vi "Histogram Test.vi"() -> ()   [LabVIEW 2012]
panel:
  out "x^y":dbl
  in  "Histogram Bin":string(combo)
  in  "Stop Delay  (ns)":i16 min=0 max=1008 step=16
  out "Waveform Graph":cluster{i16, dbl, "Array":i64[]}(graph)
  in  "Start Measurement":bool
  out "Single Count Channel4":i64
  out "Single Count Channel3":i64
  out "Single Count Channel2":i64
  out "Single Count Channel1":i64
  out "Exposition time (ms)":i64
  out "Measurement index":i64
  out "Start OK":bool
  in  "Exit":bool
  in  "Single Count Enable":T1
  in  "Channel4 Pulse Front":string
  in  "Channel4 Threshold Voltage (mV)":i32
  in  "Channel3 Pulse Front":string
  in  "Channel3 Threshold Voltage (mV)":i32
  in  "Channel2 Pulse Front":string
  in  "Channel2 Threshold Voltage (mV)":i32
  in  "Channel1 Pulse Front":string(combo)
  in  "Channel1 Threshold Voltage (mV)":i32 min=0 max=5000 step=10
  in  "Exposition Time (ms)":i64
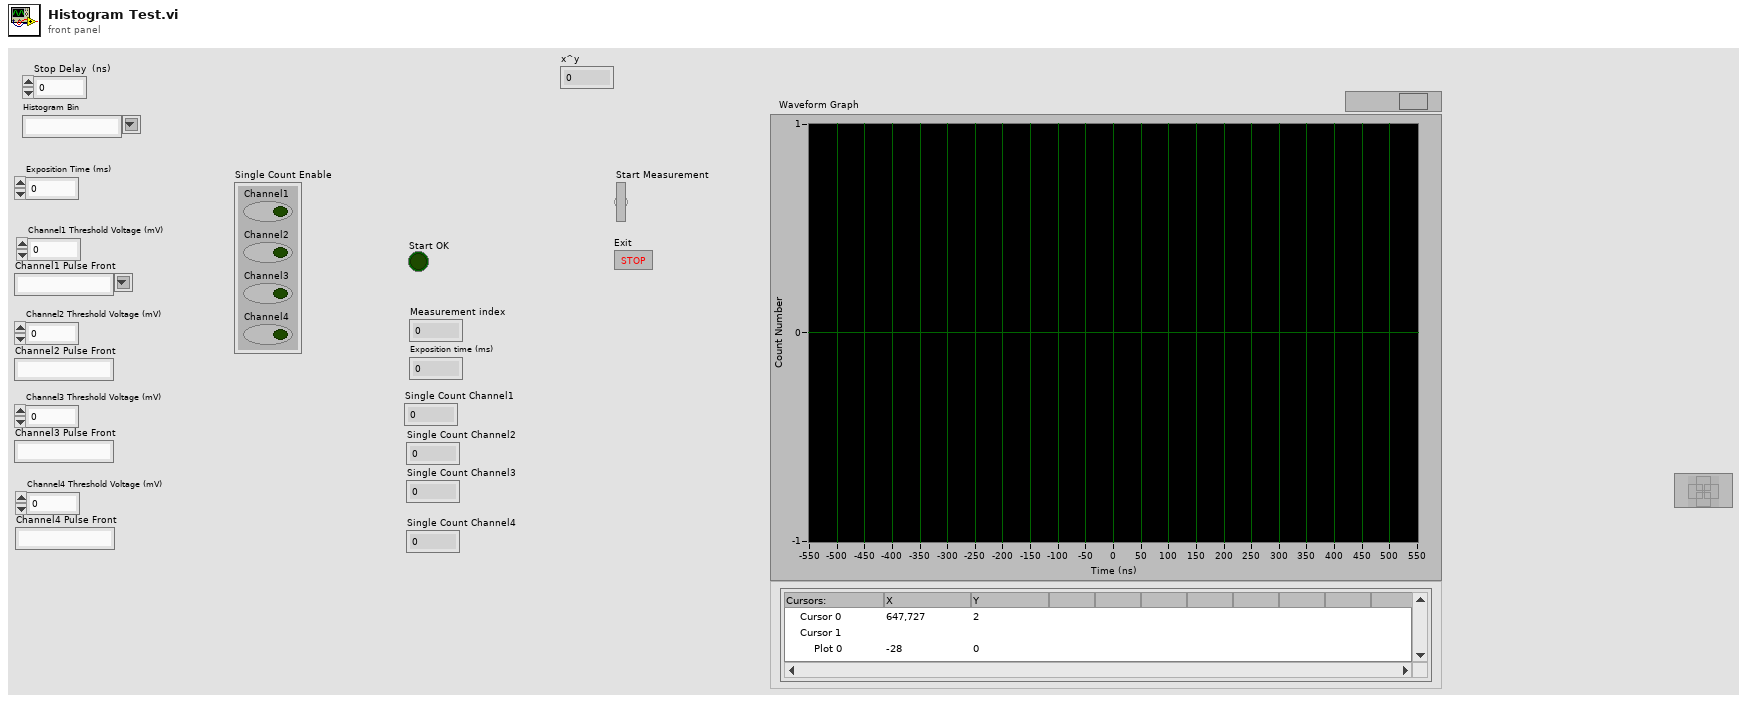
[diagram p1: front panel]
types:
  T1 = cluster{"Channel1":bool, "Channel2":bool, "Channel3":bool, "Channel4":bool}
  T2 = cluster{"[0]":i64, "Channel1 Threshold Voltage (mV)":i32, "Channel1 Pulse Front":string, "Channel2 Threshold Voltage (mV)":i32, "Channel2 Pulse Front":string, "Channel3 Threshold Voltage (mV)":i32, "Channel3 Pulse Front ":string, "Channel4 Threshold Voltage (mV)":i32, "Channel4 Pulse Front ":string, "Single Count Enable":cluster{"Channel1":bool, "Channel2":bool, "Channel3":bool, "Channel4":bool}, "Single Count Max":i32, "Sum Count Enable":cluster{"Channel1":bool, "Channel2":bool, "Channel3":bool, "Channel4":bool}, "Sum Count Max":i32, "Start-Stop1 Multyplex":cluster{"Stop Channel":string, "Start Channel":string}, "Stop Delay 1 (ns)":i16, "Window Length 1 (ns)":i32, "Window Offset 1 (ns) ":i32, "Conditional Correlation 1":string, "Histogram Bin 1":string, "Histogram Start 1 (ns) ":i32, "Start-Stop2 Multyplex ":cluster{"Stop Channel":string, "Start Channel":string}, "Stop Delay 2 (ns)":i16, "Window Length 2 (ns) ":i32, "Window Offset 2 (ns) ":i32, "Conditional Correlation 2":string, "Histogram Bin 2":string, "Histogram Start 2 (ns)  ":i32, "Start-Stop3 Multyplex":cluster{"Stop Channel":string, "Start Channel":string}, "Stop Delay 3 (ns)":i16, "Window Length 3 (ns) ":i32, "Window Offset 3 (ns) ":i32, "Conditional Correlation 3":string, "Histogram Bin 3":string, "Histogram Start 3 (ns) ":i32, "Start-Stop4 Multyplex":cluster{"Stop Channel":string, "Start Channel":string}, "Stop Delay 4 (ns)":i16, "Window Length 4 (ns)  ":i32, "Window Offset 4 (ns) ":i32, "Conditional Correlation 4":string, "Histogram Bin 4":string, "Histogram Start 4 (ns)  ":i32, "Coincidence Count Enable":cluster{"Start-Stop1":bool, "Start-Stop2":bool, "Start-Stop3":bool, "Start-Stop4":bool}, "Coincidence Count Max":i32, "Coincidence Sum Enable":cluster{"Start-Stop1":bool, "Start-Stop2":bool, "Start-Stop3":bool, "Start-Stop4":bool}, "Coincidence Sum Max":i32, "Output Channel Enable":cluster{"Channel1":bool, "Channel2":bool, "Channel3":bool, "Channel4":bool}, "Output Channel Inversion":cluster{"Channel1":bool, "Channel2":bool, "Channel3":bool, "Channel4":bool, "Output":bool}}
  T3 = cluster{"Going":bool, "Iinterrupted":bool, "Timer stop":bool, "Single count stop Ch1":bool, "Single count stop Ch2":bool, "Single count stop Ch3":bool, "Single count stop Ch4":bool, "Sum count stop":bool, "Coincidence count stop SS1":bool, "Coincidence count stop SS2":bool, "Coincidence count stop SS3":bool, "Coincidence count stop SS4":bool, "Coincidence sum count stop":bool, "Reserved":bool, "Correlator is not initialised":bool, "Internal error":bool}
  T4 = cluster{"Measurement index":i64, "Exposition time (ms)":i64, "Single Count Channel1":i64, "Single Count Channel2":i64, "Single Count Channel3":i64, "Single Count Channel4":i64, "Sum Single Count":i64, "Coincidence Count SS1":i64, "Coincidence Count SS2":i64, "Coincidence Count SS4":i64, "Coincidence Count SS5":i64, "Sum Coincidence Count":i64}
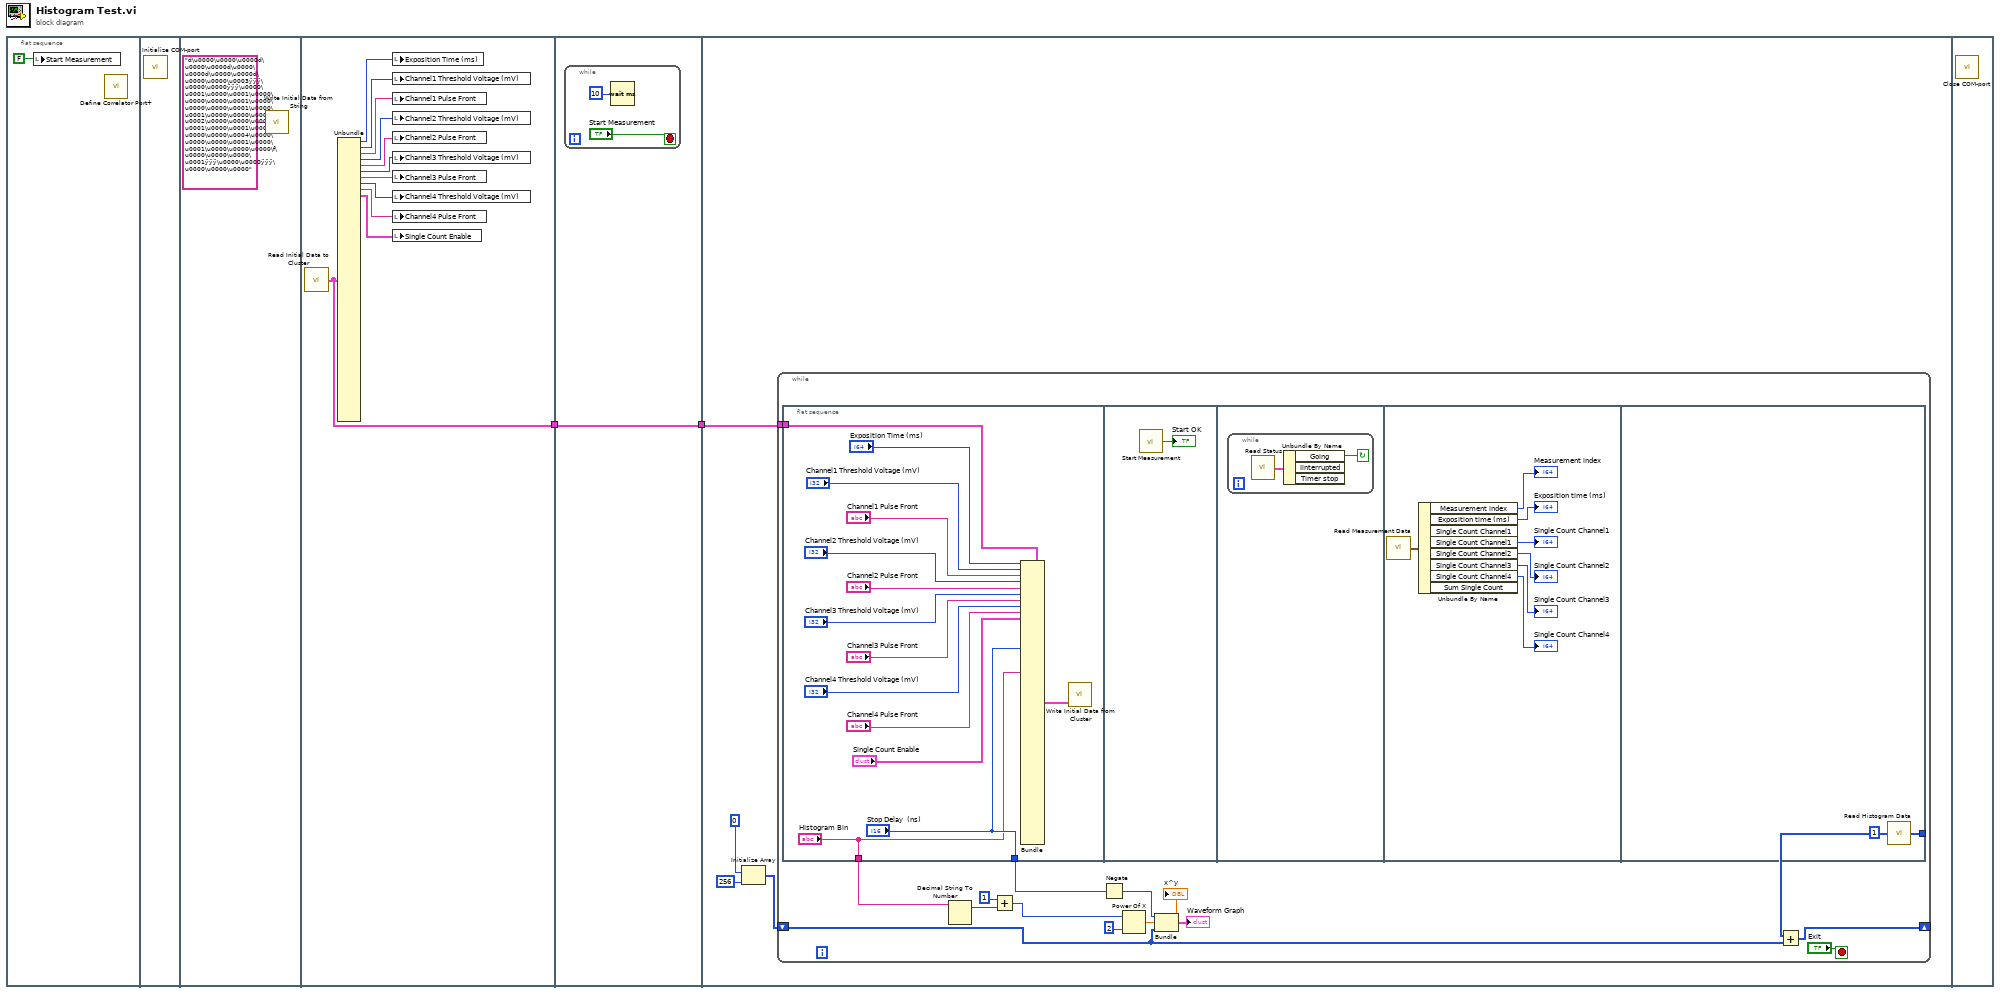
[diagram p0: block diagram]
diagram:
  n1 = flat-sequence {
    tunnel: [w15] -> w2
    tunnel: w2 -> [w16]
    tunnel: [w16] -> w1
    tunnel: w1 -> [w22]
    frame #0 {
      n2 = local write "Start Measurement"(FALSE ("Start Measurement")) -> ()
      n3 = call "Define Correlator Port+.vi"() -> ()  [unwired: 3 in]
    }
    frame #1 {
      n4 = call "Initialize COM-port.vi"() -> ()  [unwired: 4 in]
    }
    frame #2 {
      n5 = call "Write Initial Data from String.vi"("Data"="d\u0000\u0000\u0000d\u0000\u0000d\u0000\u0000d\u0000\u0000d\u0000\u0000\u0003ÿÿÿ\u0000\u0000ÿÿÿ\u0000\u0001\u0000\u0001\u0000\u0000\u0000\u0001\u0000\u0000\u0000\u0001\u0000\u0001\u0000\u0000\u0000\u0002\u0000\u0000\u0000\u0001\u0000\u0001\u0000\u0000\u0000\u0004\u0000\u0000\u0000\u0001\u0000\u0001\u0000\u0000\u0000\f\u0000\u0000\u0000\u0001ÿÿÿ\u0000\u0000ÿÿÿ\u0000\u0000\u0000") -> ()  [unwired: 1 out]
    }
    frame #3 {
      n6 = call "Read Initial Data to Cluster.vi"() -> ("Correlator Initial Data 2"=w15:T2)  [unwired: 2 in]
      n7 = Unbundle(w15) -> ("[0]"=w14:i64, "Channel1 Threshold Voltage (mV)"=w13:i32, "Channel1 Pulse Front"=w12:string, "Channel2 Threshold Voltage (mV)"=w11:i32, "Channel2 Pulse Front"=w10:string, "Channel3 Threshold Voltage (mV)"=w9:i32, "Channel3 Pulse Front"=w8:string, "Channel4 Threshold Voltage (mV)"=w7:i32, "Channel4 Pulse Front"=w6:string, "Single Count Enable"=w5:T1)  [unwired: 37 out]
      n8 = local write "Exposition Time (ms)"(w14) -> ()
      n9 = local write "Channel1 Threshold Voltage (mV)"(w13) -> ()
      n10 = local write "Channel1 Pulse Front"(w12) -> ()
      n11 = local write "Channel2 Threshold Voltage (mV)"(w11) -> ()
      n12 = local write "Channel2 Pulse Front"(w10) -> ()
      n13 = local write "Channel3 Threshold Voltage (mV)"(w9) -> ()
      n14 = local write "Channel3 Pulse Front"(w8) -> ()
      n15 = local write "Channel4 Threshold Voltage (mV)"(w7) -> ()
      n16 = local write "Channel4 Pulse Front"(w6) -> ()
      n17 = local write "Single Count Enable"(w5) -> ()
    }
    frame #4 {
      n18 = while {
        stop <- "Start Measurement" stop-if-true
        n19 = Wait (ms)(milliseconds to wait=u32 10) -> ()  [unwired: 1 out]
      }
    }
    frame #5 {
      n20 = Initialize Array(i64 0 ("Value"), 256 ("dimension size")) -> (w21:i64[])
      n21 = while {
        tunnel: w22 -> [w35]
        shift-right: [w33] -> _
        shift-left: w21 -> [w23]
        stop <- "Exit" stop-if-true
        n22 = flat-sequence {
          tunnel: w35 -> [w42]
          tunnel: ["Stop Delay  (ns)"] -> w31
          tunnel: ["Histogram Bin"] -> w29
          tunnel: [w61] -> w34
          frame #0 {
            n23 = Bundle(cluster=w42, "[0]"="Exposition Time (ms)", "Channel1 Threshold Voltage (mV)"="Channel1 Threshold Voltage (mV)", "Channel1 Pulse Front"="Channel1 Pulse Front", "Channel2 Threshold Voltage (mV)"="Channel2 Threshold Voltage (mV)", "Channel2 Pulse Front"="Channel2 Pulse Front", "Channel3 Threshold Voltage (mV)"="Channel3 Threshold Voltage (mV)", "Channel3 Pulse Front"="Channel3 Pulse Front", "Channel4 Threshold Voltage (mV)"="Channel4 Threshold Voltage (mV)", "Channel4 Pulse Front"="Channel4 Pulse Front", "Single Count Enable"="Single Count Enable", "Stop Delay 1 (ns)"="Stop Delay  (ns)", "Histogram Bin 1"="Histogram Bin") -> (w50:T2)  [unwired: 35 in]
            n24 = call "Write Initial Data from Cluster.vi"("Correlator Initial Data"=w50) -> ()  [unwired: 2 in, 1 out]
          }
          frame #1 {
            n25 = call "Start Measurement.vi"() -> ("Start OK"=→"Start OK":bool)  [unwired: 2 in]
          }
          frame #2 {
            n26 = while {
              stop <- w52 continue-if-true
              n27 = call "Read Status.vi"() -> ("Status Data"=w53:T3)  [unwired: 2 in]
              n28 = Unbundle By Name(w53) -> ("Going"=w52:bool)  [unwired: 2 out]
            }
          }
          frame #3 {
            n29 = call "Read Measurement Data.vi"() -> ("Measurement Data"=w54:T4)  [unwired: 3 in]
            n30 = Unbundle By Name(w54) -> ("Measurement index"=→"Measurement index":i64, "Exposition time (ms)"=→"Exposition time (ms)":i64, "Single Count Channel1"=→"Single Count Channel1":i64, "Single Count Channel2"=→"Single Count Channel2":i64, "Single Count Channel3"=→"Single Count Channel3":i64, "Single Count Channel4"=→"Single Count Channel4":i64)  [unwired: 2 out]
          }
          frame #4 {
            n31 = call "Read Histogram Data.vi"("Start-Stop#"=i8 1) -> ("Array"=w61:i64[])
          }
        }
        n32 = Decimal String To Number(string=w29) -> (offset past number=w28:i32)  [unwired: 2 in, 1 out]
        n33 = Add(x=1, y=w28) -> (x+y=w25:i32)
        n34 = Negate(x=w31) -> (-x=w30:i16)
        n35 = Power Of X(1:i8 2 ("x"), 2:w25) -> (0:w24:dbl)
        "x^y" <- w24
        n36 = Bundle(w30, w24, w23) -> (→"Waveform Graph":cluster{i16, dbl, i64[]})  [unwired: 1 in]
        n37 = Add(x=w34, y=w23) -> (x+y=w33:i64[])
      }
    }
    frame #6 {
      n38 = call "Close COM-port.vi"() -> ()  [unwired: 4 in]
    }
  }
